vi "Fuel Injector Section.vi"(8 "error in (no error)":errorcluster, 11 "Node Ptr":T1 format="%.0x") -> (0 "error out":errorcluster)   [LabVIEW 2015, in "Fuel Injector Analysis Addon System Explorer.lvlib"]
uses:
  Fuel Injector Analysis Addon System Explorer.lvlib
  <vilib>/NI Veristand/Custom Device API/Custom Device Item Ref.ctl
  <vilib>/NI Veristand/Custom Device API/Custom Device API.lvlib
panel:
  out "DMA Index":u16
  in  "Name":string
  in  "SHDocVw.IWebBrowser":refnum<k7>(container)
  in  "Header":cluster{"Section Name":string}={"Section Name"="Custom Device Item Settings"}
  in  "Description":string
  out "Original Name":string
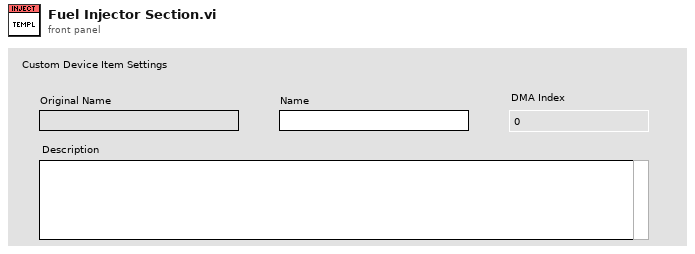
[diagram p1: front panel]
types:
  T1 = typedef "Custom Device API.lvlib/Custom Device Item Ref.ctl" = u64
  T2 = typedef "Custom Device API.lvlib/Custom Device Item Info.ctl" = cluster{"Name":string, "Is Channel":bool, "GUID":string, "Is Waveform":bool}
  T3 = typedef "Custom Device API.lvlib/Custom Device Commands.ctl" = enum16{"Default", "Item renamed", "Shutdown", "Dynamic button pressed"}
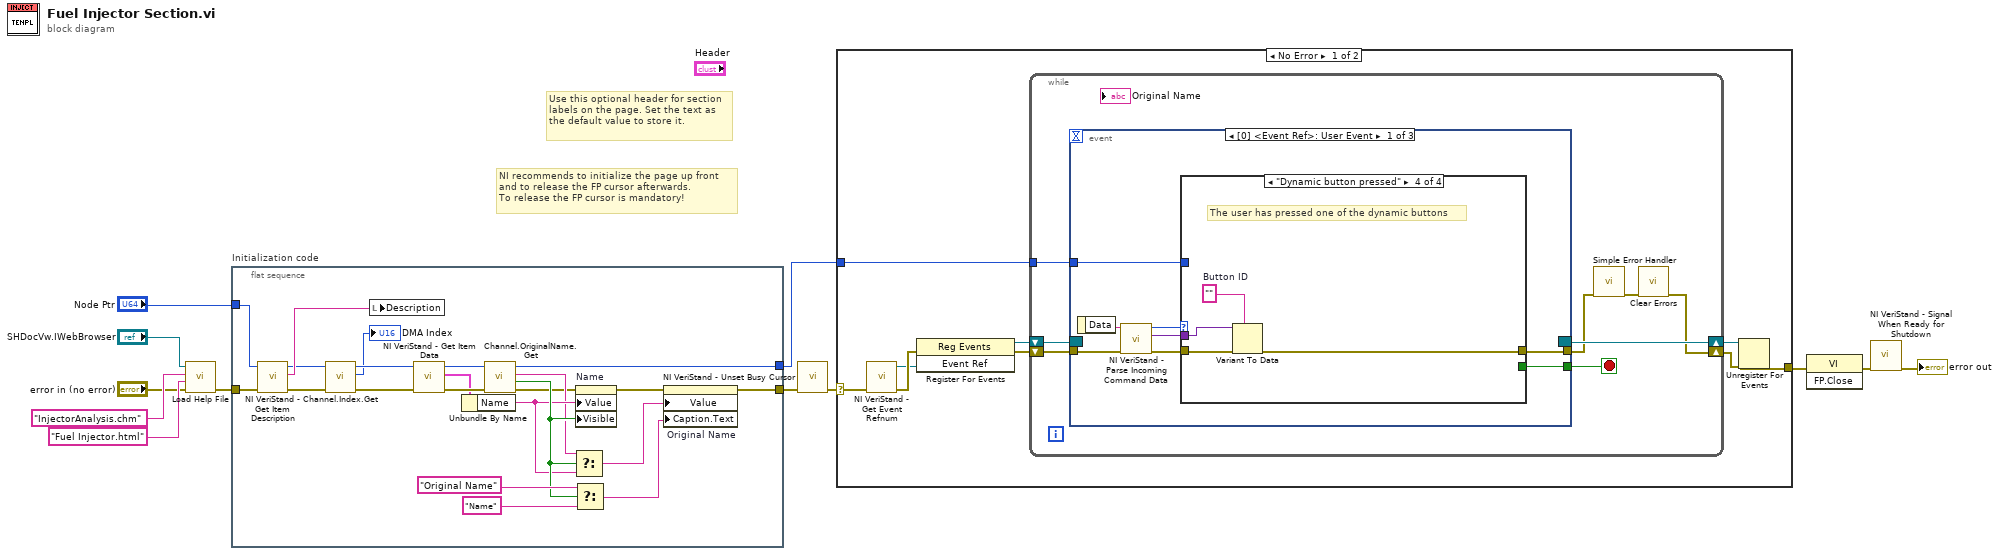
[diagram p0: block diagram]
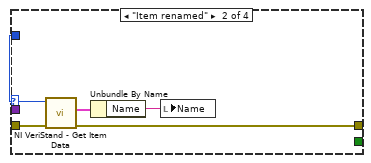
[diagram p3: hidden frame]
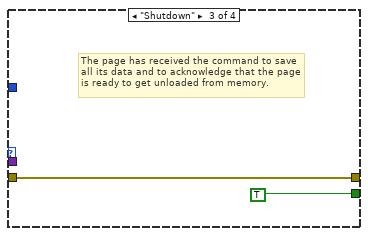
[diagram p4: hidden frame]
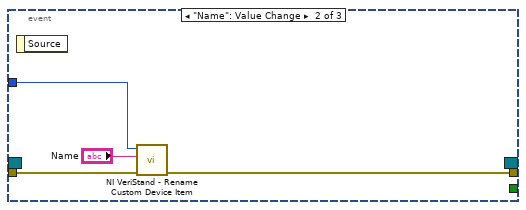
[diagram p5: hidden frame]
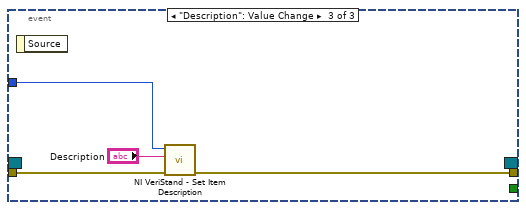
[diagram p6: hidden frame]
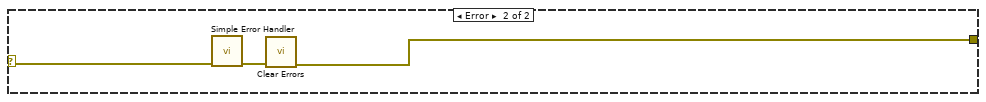
[diagram p7: hidden frame]
diagram:
  # "Use this optional header for section labels on the page. Set the text as the default value to store it."
  # "NI recommends to initialize the page up front\nand to release the FP cursor afterwards.\nTo release the FP cursor is mandatory!"
  n1 = call "Load Help File.vi"("error in (no error)"="error in (no error)", "HTML File"="Fuel Injector.html", "Main CHM File"="InjectorAnalysis.chm", "SHDocVw.IWebBrowser2"="SHDocVw.IWebBrowser") -> ("error out"=w3:errorcluster)  [unwired: 7 in]
  n2 = flat-sequence "Initialization code" {
    tunnel: w3 -> [w34]
    tunnel: [w19] -> w9
    tunnel: [w18] -> w7
    tunnel: "Node Ptr" -> [w32]
    frame #0 {
      n3 = call <vilib>:"NI VeriStand - Get Item Description.vi"("error in (no error)"=w34, "Item Ref in"=w32) -> ("error out"=w16:errorcluster, "Description"=w33:string, "Item Ref out"=w17:T1)  [unwired: 7 out]
      n4 = call "Channel.Index.Get.vi"("error in (no error)"=w16, "Ref in"=w17) -> ("error out"=w14:errorcluster, "Value"=→"DMA Index":u16, "Ref out"=w15:T1)  [unwired: 6 in, 1 out]
      n5 = local write "Description"(w33) -> ()
      n6 = call <vilib>:"NI VeriStand - Get Item Data.vi"("error in (no error)"=w14, "Item Ref in"=w15) -> ("error out"=w22:errorcluster, "Item Info"=w20:T2, "Item Ref out"=w21:T1)  [unwired: 7 out]
      n7 = Unbundle By Name(w20) -> ("Name"=w26:string)
      n8 = call "Channel.OriginalName.Get.vi"("error in (no error)"=w22, "Ref in"=w21) -> ("error out"=w23:errorcluster, "Found?"=w28:bool, "Value"=w25:string, "Ref out"=w18:T1)  [unwired: 6 in]
      n9 = Select(t=w25, s=w28, f=w26) -> (s? t:f=w27:string)
      n10 = Select(t="Original Name" ("s? t:f"), s=w28, f="Name" ("s? t:f")) -> (s? t:f=w31:string)
      n11 = property on="Name" class="Str"(error in=w23, "Value"=w26, "Visible"=w28) -> (error out=w24:errorcluster)  [unwired: 1 in, 1 out]
      n12 = property on="Original Name" class="Str"(error in=w24, "Value"=w27, "Caption.Text"=w31) -> (error out=w19:errorcluster)  [unwired: 1 in, 1 out]
    }
  }
  n13 = call <vilib>:"NI VeriStand - Unset Busy Cursor.vi"("error in (no error)"=w9) -> ("error out"=w8:errorcluster)  [unwired: 10 out]
  n14 = case shown="No Error" w8 {
    selector: w8 -> [w35 w82]
    tunnel: [w40 w80] -> w12
    tunnel: w7 -> [w36 _]
    frame No Error {
      n15 = call <vilib>:"NI VeriStand - Get Event Refnum.vi"("error in (no error)"=w35) -> ("error out"=w43:errorcluster, "Event Ref"=w39:refnum<user-event>)  [unwired: 9 out]
      n16 = register-events(error in=w43, w39) -> (reference out=w37:refnum<event-registration>, error out=w38:errorcluster)  [unwired: 1 in]
      n17 = while {
        tunnel: w36 -> [w47]
        shift-right: [w44] -> w41
        shift-left: w38 -> [w50]
        shift-right: [w51] -> w42
        shift-left: w37 -> [w49]
        stop <- w48 stop-if-true
        n18 = event shown="[0] <Event Ref>: User Event" {
          selector: w49 -> [_ _ _]
          dyn-events: [_ _ _] -> w51
          timeout: _ -> [_ _ _]
          tunnel: w50 -> [w59 w75 w78]
          tunnel: [w55 _ _] -> w48
          tunnel: [w54 w74 w77] -> w46
          tunnel: w47 -> [w53 w73 w79]
          event User Event {
            n19 = event-data() -> ("Data"=w58:string)  [unwired: 1 out]
            n20 = call <vilib>:"NI VeriStand - Parse Incoming Command Data.vi"("error in (no error)"=w59, "Incoming data"=w58) -> ("error out"=w57:errorcluster, "Outgoing data"=w52:variant, "Action"=w56:T3)  [unwired: 7 out]
            n21 = case shown="\"Dynamic button pressed\"" w56 {
              tunnel: w57 -> [w60 w65 w66 w71]
              tunnel: [_ _ TRUE _] -> w55
              tunnel: [w60 w63 w66 w68] -> w54
              tunnel: w53 -> [_ w64 _ _]
              tunnel: w52 -> [_ _ _ w70]
              frame "Default", Default {
              }
              frame "Item renamed" {
                n22 = call <vilib>:"NI VeriStand - Get Item Data.vi"("error in (no error)"=w65, "Item Ref in"=w64) -> ("error out"=w63:errorcluster, "Item Info"=w62:T2)  [unwired: 8 out]
                n23 = Unbundle By Name(w62) -> ("Name"=w61:string)
                n24 = local write "Name"(w61) -> ()
              }
              frame "Shutdown" {
                # "The page has received the command to save all its data and to acknowledge that the page is ready to get unloaded from memory."
              }
              frame "Dynamic button pressed" {
                w69 = ""  # Button ID
                # "The user has pressed one of the dynamic buttons"
                n25 = Variant To Data(error in=w71, type=w69, Variant=w70) -> (error out=w68:errorcluster)  [unwired: 1 out]
              }
            }
          }
          event "Name": Value Change {
            n26 = event-data() -> ()  [unwired: 2 out]
            n27 = call <vilib>:"NI VeriStand - Rename Custom Device Item.vi"("error in (no error)"=w75, "New Name"="Name", "Item Ref in"=w73) -> ("error out"=w74:errorcluster)  [unwired: 1 in, 7 out]
          }
          event "Description": Value Change {
            n28 = event-data() -> ()  [unwired: 2 out]
            n29 = call <vilib>:"NI VeriStand - Set Item Description.vi"("error in (no error)"=w78, "Description"="Description", "Item Ref in"=w79) -> ("error out"=w77:errorcluster)  [unwired: 8 out]
          }
        }
        n30 = call <vilib>:"Simple Error Handler.vi"("error in (no error)"=w46) -> ("error out"=w45:errorcluster)  [unwired: 1 in, 7 out]
        n31 = call <vilib>:"Clear Errors.vi"("error in (no error)"=w45) -> ("error out"=w44:errorcluster)  [unwired: 1 in, 5 out]
      }
      n32 = Unregister For Events(event registration refnum=w42, error in=w41) -> (error out=w40:errorcluster)
    }
    frame Error {
      n33 = call <vilib>:"Simple Error Handler.vi"("error in (no error)"=w82) -> ("error out"=w81:errorcluster)  [unwired: 1 in, 7 out]
      n34 = call <vilib>:"Clear Errors.vi"("error in (no error)"=w81) -> ("error out"=w80:errorcluster)  [unwired: 1 in, 5 out]
    }
  }
  n35 = invoke class="VI" method="FP.Close"(error in=w12) -> (error out=w11:errorcluster)  [unwired: 2 in, 2 out]
  n36 = call <vilib>:"NI VeriStand - Signal When Ready for Shutdown.vi"("error in (no error)"=w11) -> ("error out"=→"error out":errorcluster)  [unwired: 10 out]
